vi "Get Scan Engine Mode.vi"(8 "error in (no error)":errorcluster, 11 "target address (localhost)":string="localhost") -> (0 "error out":errorcluster, 2 "mode":i32(ring)=2 items=["Initialization Mode", "Configuration Mode", "Active Mode", "Fault Mode"])   [LabVIEW 2020]
doc: "Returns the operating mode of the NI Scan Engine on the target."
uses:
  <resource>/objmgr/ni.var.rc
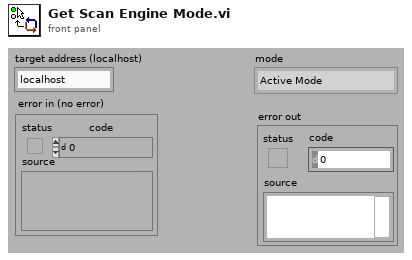
[diagram p1: front panel]
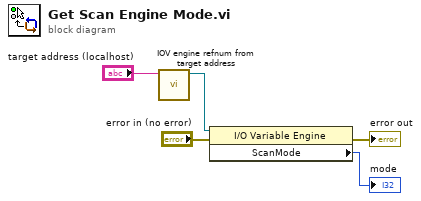
[diagram p0: block diagram]
diagram:
  n1 = call <vilib>:"IOV engine refnum from target address.vi"("target address"="target address (localhost)") -> ("reference out"=w4:refnum<k21>)  [unwired: 10 in]
  n2 = property class="I/O Variable Engine"(reference=w4, error in="error in (no error)") -> (error out=→"error out":errorcluster, "ScanMode"=→"mode":i32)  [unwired: 1 out]
